vi "Subvi digital delay.vi"(8 "Delay_tick":u32, 10 "Input":bool) -> (2 "Output":bool)   [LabVIEW 2017]
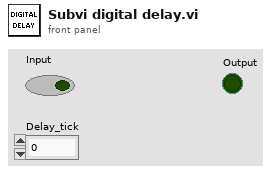
[diagram p1: front panel]
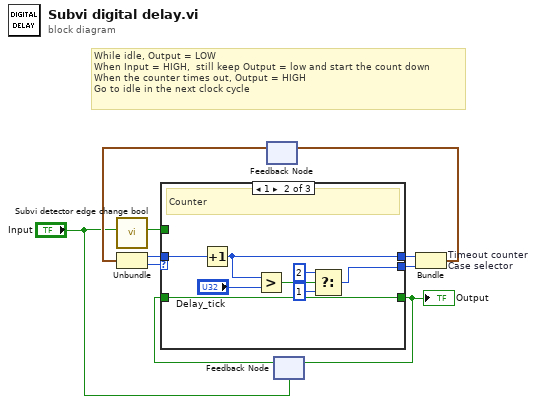
[diagram p0: block diagram]
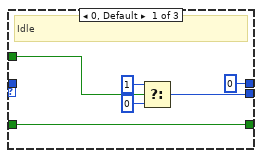
[diagram p2: hidden frame]
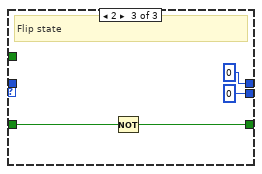
[diagram p3: hidden frame]
diagram:
  # "While idle, Output = LOW\nWhen Input = HIGH,  still keep Output = low and start the count down\nWhen the counter times out, Output = HIGH\nGo to idle in the next clock cycle"
  n1 = call "Subvi detector edge change bool.vi"("Input"="Input") -> ("Output"=w10:bool)  [unwired: 8 in]
  n2 = feedback #1() -> (w6:cluster{u32, "f":u8})  [unwired: 1 in]
  n3 = Unbundle(w6) -> (w5:u32, "f"=w4:u8)
  n4 = feedback #2("Input") -> (w3:bool)
  n5 = case shown="1" w4 {
    tunnel: [w15 w20 w27] -> w1
    tunnel: [u32 0 w22 u32 0] -> w9
    tunnel: w5 -> [_ w23 _]
    tunnel: w3 -> [w15 w20 w28]
    tunnel: [w12 w19 u8 0 ("f")] -> w8
    tunnel: w10 -> [w11 _ _]
    frame 0, Default {
      # "Idle"
      n6 = Select(t=u8 1, s=w11, f=u8 0) -> (s? t:f=w12:u8)
    }
    frame 1 {
      # "Counter"
      n7 = Increment(x=w23) -> (x+1=w22:u32)
      n8 = Greater?(x=w22, y="Delay_tick") -> (0:w24:bool)
      n9 = Select(t=u8 2, s=w24, f=u8 1) -> (s? t:f=w19:u8)
    }
    frame 2 {
      # "Flip state"
      n10 = Not(x=w28) -> (.not. x?=w27:bool)
    }
  }
  "Output" <- w1
  n11 = feedback-in #2(w1) -> ()
  n12 = Bundle "Timeout counter\nCase selector"(w9, "f"=w8) -> (w7:cluster{u32, "f":u8})  [unwired: 1 in]
  n13 = feedback-in #1(w7) -> ()
